vi "TCP Factory.vi"(8 "Error In":errorcluster, 10 "TCP Settings":T1) -> (0 "Error Out":errorcluster, 3 "TCP Out":refnum<class "TCP.lvclass">)   [LabVIEW 2018, in "Protocols.lvlib" / "TCP.lvclass"]
doc: "Instantiates a new TCP Protocol object using the provided TCP Settings\n\nInput: \nTCP Settings:\n IP Address: specifies the IP Address of the system with which you want to establish a connection.\n Port: it's the Port of the service with which you want to establish a connection.\n\nOutput: \nTCP Object created using the provided TCP Settings"
uses:
  TCP.lvclass
  TCP Settings.ctl
  TCP.lvclass/TCP.ctl
  Data Access/Write IP Address.vi
  Data Access/Write Port.vi
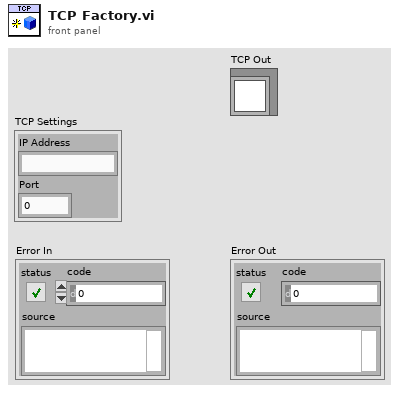
[diagram p1: front panel]
types:
  T1 = typedef "Protocols.lvlib/TCP.lvclass/TCP Settings.ctl" = cluster{"IP Address":string, "Port":u16}
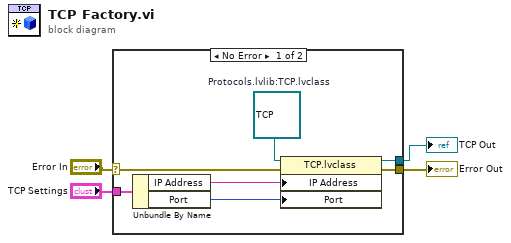
[diagram p0: block diagram]
diagram:
  n1 = case shown="No Error" "Error In" {
    selector: "Error In" -> [w5 w12]
    tunnel: "TCP Settings" -> [w11 _]
    tunnel: [w7 _] -> w3
    tunnel: [w6 w12] -> w2
    frame No Error {
      w10 = refnum<class "TCP.lvclass"> refnum  # Protocols.lvlib:TCP.lvclass
      n2 = Unbundle By Name(w11) -> ("IP Address"=w9:string, "Port"=w8:u16)
      n3 = property class="TCP.lvclass"(reference=w10, error in=w5, "IP Address"=w9, "Port"=w8) -> (reference out=w7:refnum<class "TCP.lvclass">, error out=w6:errorcluster)
    }
    frame Error {
    }
  }
  "TCP Out" <- w3
  "Error Out" <- w2
